vi "GetLatestVersion.vi"() -> (2 "LastVersion":T1)   [LabVIEW 2017]
uses:
  <vilib>/AppBuilder/AB_API_Simple/Build Specification Version.ctl
  <vilib>/AppBuilder/AB_API_Simple/NI_App_Builder_API.lvlib
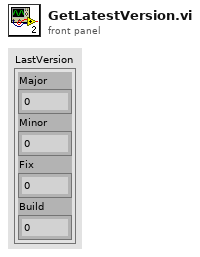
[diagram p1: front panel]
types:
  T1 = typedef "NI_App_Builder_API.lvlib/Build Specification Version.ctl" = cluster{"Major":u16, "Minor":u16, "Fix":u16, "Build":u16}
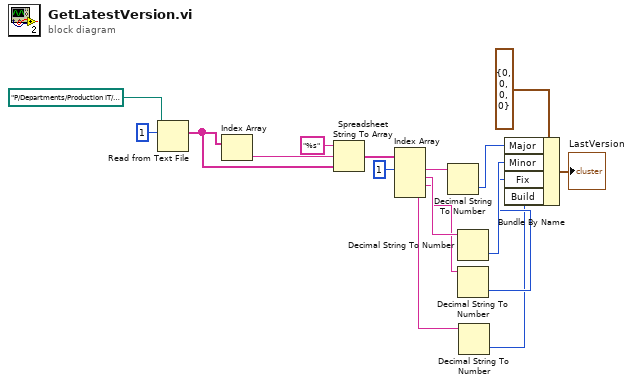
[diagram p0: block diagram]
diagram:
  n1 = Read from Text File(file (use dialog)=path "P:/Departments/Production IT/Software/GVS/BetaTest_NOT_FOR_PRODUCTION/.metadata/release info.txt", count=1) -> (text=w14:string[])  [unwired: 2 in, 3 out]
  n2 = Index Array(array=w14) -> (element=w15:string)  [unwired: 1 in]
  n3 = Spreadsheet String To Array(format string="%s", spreadsheet string=w15, array type (2D Dbl)=w14) -> (array=w13:string[])  [unwired: 1 in]
  n4 = Index Array(array=w13, index #1=1 ("index")) -> (element #1=w9:string, element #2=w8:string, element #3=w7:string, element #4=w3:string)  [unwired: 3 in]
  n5 = Decimal String To Number(string=w9) -> (number=w6:i32)  [unwired: 2 in, 1 out]
  n6 = Decimal String To Number(string=w8) -> (number=w5:i32)  [unwired: 2 in, 1 out]
  n7 = Decimal String To Number(string=w7) -> (number=w4:i32)  [unwired: 2 in, 1 out]
  n8 = Decimal String To Number(string=w3) -> (number=w2:i32)  [unwired: 2 in, 1 out]
  n9 = Bundle By Name(cluster=T1 {"Major"=0, "Minor"=0, "Fix"=0, "Build"=0} ("Build Specification Version"), "Major"=w6, "Minor"=w5, "Fix"=w4, "Build"=w2) -> (→"LastVersion":T1)
